vi "checksf.vi"() -> ()   [LabVIEW 2011]
uses:
  global.vi
panel:
  out "Received data from mote":string
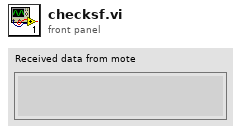
[diagram p1: front panel]
types:
  T1 = enum16{"open", "replace", "create", "open or create", "replace or create", "replace or create with confirmation"}
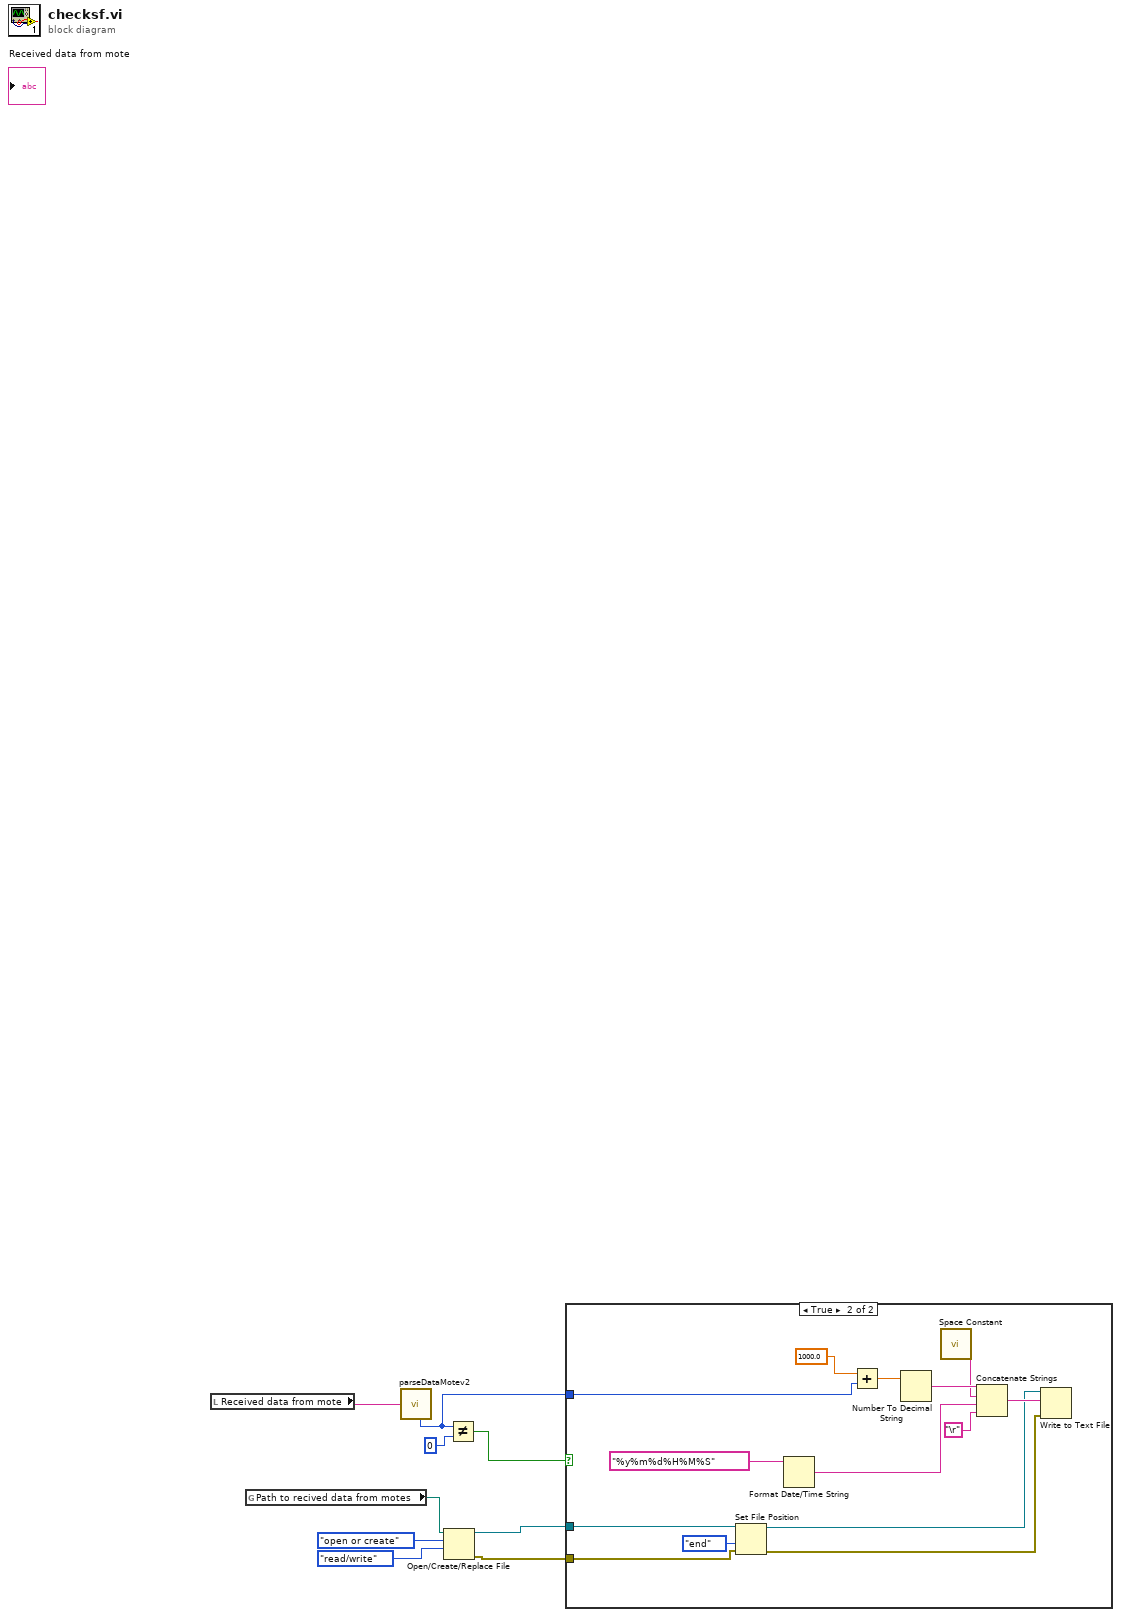
[diagram p0: block diagram]
diagram:
  n1 = local read "Received data from mote"() -> (w6:string)
  n2 = global read "global.vi" "Path to recived data from motes"() -> (w3:path)
  n3 = call "parseDataMotev2.vi"("input data"=w6) -> ("node id (1 byte)"=w9:u8)  [unwired: 5 out]
  n4 = Open/Create/Replace File(file path (use dialog)=w3, operation (0:open)=T1."open or create", access (0:read/write)=enum16{"read/write", "read-only", "write-only"}."read/write") -> (refnum out=w4:refnum<file>, error out=w5:errorcluster)  [unwired: 3 in, 1 out]
  n5 = Not Equal?(x=w9, y=u8 0) -> (x != y?=w8:bool)
  n6 = case shown="True" w8 {
    tunnel: w4 -> [_ w23]
    tunnel: w5 -> [_ w22]
    tunnel: w9 -> [_ w10]
    frame False {
    }
    frame True {
      n7 = Set File Position(refnum=w23, from (0:start)=enum16{"start", "end", "current"}."end", error in=w22) -> (refnum out=w12:refnum<file>, error out=w11:errorcluster)  [unwired: 1 in]
      n8 = Format Date/Time String(time format string (%c)="%y%m%d%H%M%S") -> (date/time string=w16:string)  [unwired: 2 in]
      n9 = Add(x=1000.0 ("y"), y=w10) -> (x+y=w19:dbl)
      n10 = Number To Decimal String(number=w19) -> (decimal integer string=w18:string)  [unwired: 1 in]
      n11 = call <vilib>:"Space Constant.vi"() -> ("String"=w17:string)
      n12 = Concatenate Strings(w18, w17, w16, "\r") -> (w14:string)
      n13 = Write to Text File(file (use dialog)=w12, text=w14, error in=w11) -> ()  [unwired: 1 in, 3 out]
    }
  }
